vi "Bool to TF.vi"(1 "Boolean":bool=TRUE) -> (0 "T/F":string)   [LabVIEW 2016]
doc: "Turns a True/False boolean value into a T/F string."
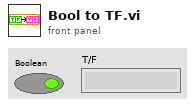
[diagram p1: front panel]
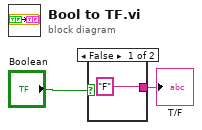
[diagram p0: block diagram]
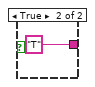
[diagram p2: hidden frame]
diagram:
  n1 = case shown="False" "Boolean" {
    tunnel: ["F" "T"] -> w1
    frame False {
    }
    frame True {
    }
  }
  "T/F" <- w1
